vi "Z6_Beamline.set States in GUI.vi"(0 "i ref in":refnum<vi>, 5 "error in":errorcluster) -> (14 "i ref out":refnum<vi>, 19 "error out":errorcluster)   [LabVIEW 2014, in "Z6_Beamline.lvlib"]
uses:
  Z6_Beamline.lvlib
  PH_BL-Master/PH_BL-Master.lvlib
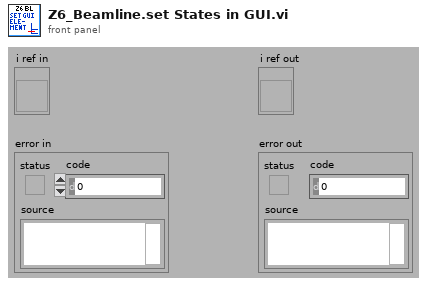
[diagram p1: front panel]
types:
  T1 = typedef "PH_BL-Master.lvlib/PH_BL-Master.i attribute.ctl" = cluster{"Remote controlled":bool, "Boolean Condition Service Subscriber":refnum<vi>[], "Picture Condition Service Subscriber":refnum<vi>[], "R2S":cluster{"GUI Ref":refnum<vi>, "State":bool}, "Vacua":cluster{"GUI Ref":refnum<vi>, "Limit":dbl, "Curr Value":dbl, "in range":bool}[], "O2 Inspection":cluster{"GUI Ref":refnum<vi>, "Concentration":dbl, "State":T2}[], "Boolean Status Service Subscriber":cluster{"GUI Ref":refnum<vi>, "Status":T2, "no Link?":bool, "Status Subscriber Class":T3}[], "Picture Status Service Subscriber":cluster{"GUI Ref":refnum<vi>, "Status":T2, "no Link?":bool, "Status Subscriber Class":T3}[], "6P 4Q Service Subscriber":cluster{"GUI Ref":refnum<vi>, "Selector":T4, "no Link?":bool}[], "Index of latest 6P 4Q changing Instance":i32, "Index of latest Picture Status changing Instance":i32, "Index of latest Boolean Status changing Instance":i32, "Vision ID on same Node":string, "Start Phase over?":bool, "GUI Ref Delete":refnum<vi>}
  T2 = typedef "PH_StatusHandler.lvlib/PH_StatusHandler.Status.ctl" = i16
  T3 = typedef "PH_BL-Master.lvlib/PH_BL-Master.Status Subscriber Class.ctl" = enum16{"unknown", "Switch", "BB", "6P Switch", "Switch GUI", "Switch and 6P State", "Force Sensor"}
  T4 = typedef "PH_4_Pos_Selector.lvlib/PH_4_Pos_Selector.Position Selector.ctl" = u16
  T5 = cluster{"GUI Ref":refnum<vi>, "Status":T2, "no Link?":bool, "Status Subscriber Class":T3}[]
  T6 = cluster{"GUI Ref":refnum<vi>, "Status":T2, "no Link?":bool, "Status Subscriber Class":T3}
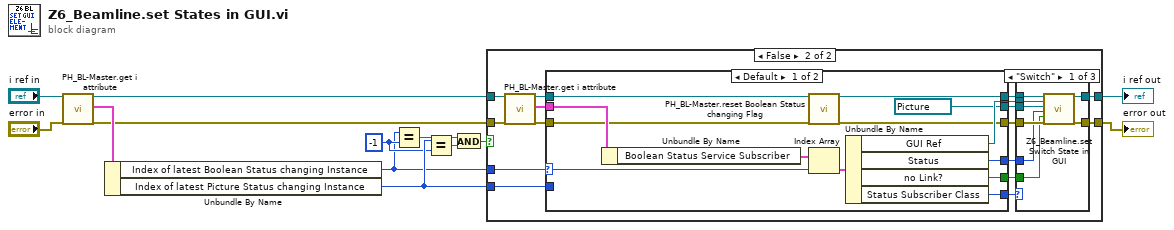
[diagram p0: block diagram]
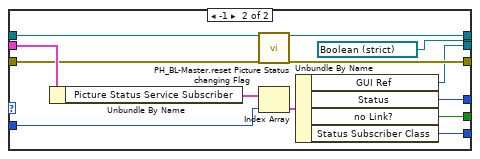
[diagram p3: hidden frame]
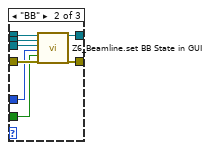
[diagram p4: hidden frame]
diagram:
  w5 = -1 ("y")
  n1 = call "PH_BL-Master.get i attribute.vi"("i ref in"="i ref in", "error in (no error)"="error in") -> ("i ref out"=w12:refnum<vi>, "i attribute"=w13:T1, "error out"=w10:errorcluster)  [unwired: 15 in]
  n2 = Unbundle By Name(w13) -> ("Index of latest Boolean Status changing Instance"=w2:i32, "Index of latest Picture Status changing Instance"=w6:i32)
  n3 = Equal?(x=w2, y=w5) -> (x = y?=w4:bool)
  n4 = Equal?(x=w6, y=w5) -> (x = y?=w3:bool)
  n5 = And(x=w4, y=w3) -> (x .and. y?=w1:bool)
  n6 = case shown="False" w1 {
    tunnel: [w15 w24] -> w7
    tunnel: [w14 w23] -> w9
    tunnel: w10 -> [w14 w31]
    tunnel: w12 -> [w15 w30]
    tunnel: w6 -> [_ w17]
    tunnel: w2 -> [_ w16]
    frame True {
    }
    frame False {
      n7 = call "PH_BL-Master.get i attribute.vi"("i ref in"=w30, "error in (no error)"=w31) -> ("i ref out"=w20:refnum<vi>, "i attribute"=w29:T1, "error out"=w22:errorcluster)  [unwired: 15 in]
      n8 = case shown="Default" w16 {
        selector: w16 -> [w32 _]
        tunnel: w29 -> [w44 w57]
        tunnel: [w41 w56] -> w28
        tunnel: [w40 w55] -> w27
        tunnel: [w39 w54] -> w26
        tunnel: [w38 refnum<vi> refnum ("GUI Ref")] -> w25
        tunnel: w22 -> [w37 w52]
        tunnel: [w36 w51] -> w21
        tunnel: w20 -> [w35 w50]
        tunnel: [w34 w49] -> w19
        tunnel: [refnum<vi> refnum ("Pic GUI Ref") w48] -> w18
        tunnel: w17 -> [_ w47]
        frame Default {
          n9 = Unbundle By Name(w44) -> ("Boolean Status Service Subscriber"=w43:T5)
          n10 = call "PH_BL-Master.reset Boolean Status changing Flag.vi"("i ref in"=w35, "error in"=w37) -> ("i ref out"=w34:refnum<vi>, "error out"=w36:errorcluster)  [unwired: 16 in]
          n11 = Index Array(array=w43, index=w32) -> (element=w42:T6)
          n12 = Unbundle By Name(w42) -> ("GUI Ref"=w38:refnum<vi>, "Status"=w39:T2, "no Link?"=w40:bool, "Status Subscriber Class"=w41:T3)
        }
        frame -1 {
          n13 = Unbundle By Name(w57) -> ("Picture Status Service Subscriber"=w46:T5)
          n14 = call "PH_BL-Master.reset Picture Status changing Flag.vi"("i ref in"=w50, "error in"=w52) -> ("i ref out"=w49:refnum<vi>, "error out"=w51:errorcluster)  [unwired: 16 in]
          n15 = Index Array(array=w46, index=w47) -> (element=w45:T6)
          n16 = Unbundle By Name(w45) -> ("GUI Ref"=w48:refnum<vi>, "Status"=w54:T2, "no Link?"=w55:bool, "Status Subscriber Class"=w56:T3)
        }
      }
      n17 = case shown="\"Switch\"" w28 {
        tunnel: [w64 w73 w75] -> w24
        tunnel: [w62 w72 w74] -> w23
        tunnel: w21 -> [w63 w71 w74]
        tunnel: w19 -> [w65 w70 w75]
        tunnel: w27 -> [w61 w66 _]
        tunnel: w26 -> [w60 w67 _]
        tunnel: w25 -> [w59 w69 _]
        tunnel: w18 -> [w58 w68 _]
        frame "Switch" {
          n18 = call "Z6_Beamline.set Switch State in GUI.vi"("i ref in"=w65, "Boolean GUI Ref"=w59, "Pic GUI Ref"=w58, "Status"=w60, "no Link?"=w61, "error in (no error)"=w63) -> ("i ref out"=w64:refnum<vi>, "error out"=w62:errorcluster)  [unwired: 12 in]
        }
        frame "BB" {
          n19 = call "Z6_Beamline.set BB State in GUI.vi"("i ref in"=w70, "Boolean GUI Ref"=w69, "Pic GUI Ref"=w68, "State Status"=w67, "no Link?"=w66, "error in"=w71) -> ("i ref out"=w73:refnum<vi>, "error out"=w72:errorcluster)  [unwired: 12 in]
        }
        frame Default {
        }
      }
    }
  }
  "error out" <- w9
  "i ref out" <- w7
